vi "UDP Discover.vi"(0 "Name":string, 11 "error in (no error)":errorcluster) -> (4 "address:port":string, 6 "Address":string, 8 "Port":i32, 10 "format":string, 15 "error out":errorcluster)   [LabVIEW 2020]
uses:
  <vilib>/Utility/tcp.llb/UDP Multicast Read-Write Open.vi
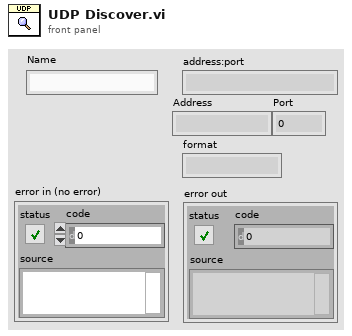
[diagram p1: front panel]
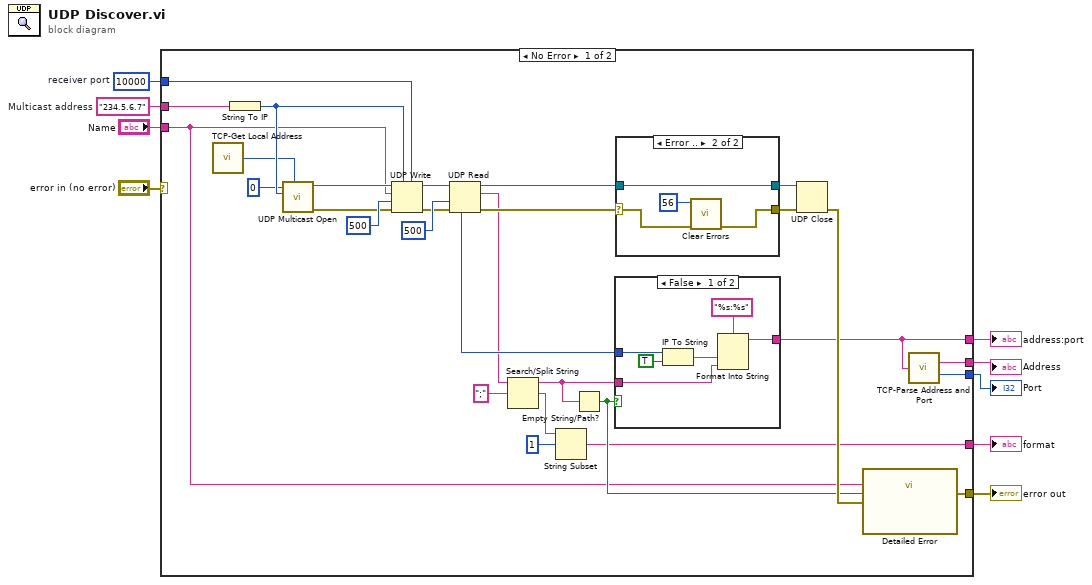
[diagram p0: block diagram]
diagram:
  w8 = u16 10000  # receiver port
  w9 = "234.5.6.7"  # Multicast address
  n1 = case shown="No Error" "error in (no error)" {
    selector: "error in (no error)" -> [_ w51]
    tunnel: w9 -> [w38 _]
    tunnel: w8 -> [w37 _]
    tunnel: [w18 _] -> w7
    tunnel: "Name" -> [w21 _]
    tunnel: [w20 w51] -> w5
    tunnel: [w17 _] -> w3
    tunnel: [w16 _] -> w2
    tunnel: [w10 _] -> w1
    frame No Error {
      n2 = call "TCP-Get Local Address.vi"() -> ("net address"=w19:u32)  [unwired: 14 in, 1 out]
      n3 = String To IP(1:w38) -> (0:w36:u32)
      n4 = call-poly <vilib>:"UDP Multicast Open.vi"("net address"=w19, "multicast addr"=w36, "port"=u16 0) -> ("error out"=w33:errorcluster, "connection ID"=w32:refnum<k16>)  [unwired: 6 in, 1 out]
      n5 = UDP Write(address=w36, port or service name=w37, connection ID=w32, data in=w21, 8:w33, 9:500 ("timeout ms (25000)")) -> (error out=w29:errorcluster, 3:w26:refnum<k16>)
      n6 = UDP Read(connection ID=w26, timeout ms (25000)=500, 8:w29) -> (data out=w15:string, error out=w27:errorcluster, 3:w25:refnum<k16>, 6:w24:u32)  [unwired: 2 out]
      n7 = Search/Split String(string=w15, search string/char (-)=";") -> (substring before match=w13:string, match + rest of string=w12:string)  [unwired: 1 in, 1 out]
      n8 = String Subset(string=w12, offset (0)=1) -> (substring=w10:string)  [unwired: 1 in]
      n9 = Empty String/Path?(string/path=w13) -> (empty?=w22:bool)
      n10 = case shown="False" w22 {
        tunnel: w24 -> [w44 _]
        tunnel: [w40 _] -> w18
        tunnel: w13 -> [w39 _]
        frame False {
          n11 = IP To String(1:TRUE ("dot notation? (F)"), 2:w44) -> (0:w42:string)
          n12 = Format Into String(format string="%s:%s", w42, w39) -> (resulting string=w40:string)  [unwired: 2 in, 1 out]
        }
        frame True {
        }
      }
      n13 = case shown="Error .." w27 {
        selector: w27 -> [w45 w48]
        tunnel: w25 -> [w46 w50]
        tunnel: [w46 w50] -> w31
        tunnel: [w45 w47] -> w30
        frame No Error {
        }
        frame Error {
          n14 = call <vilib>:"Clear Errors.vi"("error in (no error)"=w48, "specific error code to clear (0: all)"=56) -> ("error out"=w47:errorcluster)  [unwired: 4 in, 1 out]
        }
      }
      n15 = UDP Close(connection ID=w31, 8:w30) -> (error out=w23:errorcluster)  [unwired: 1 out]
      n16 = call "Detailed Error"("Details"=w21, "Error?"=w22, "Primary"=w23) -> ("detailed error"=w20:errorcluster)  [unwired: 12 in]
      n17 = call "TCP-Parse Address and Port.vi"("Address in"=w18) -> ("Address"=w17:string, "Port"=w16:i32)  [unwired: 12 in, 1 out]
    }
    frame Error {
    }
  }
  "address:port" <- w7
  "error out" <- w5
  "Address" <- w3
  "Port" <- w2
  "format" <- w1
